vi "Firmware Wizard.vi"() -> ()   [LabVIEW 2011, in "LMH-LINX.lvlib"]
doc: "Wizard for uploading firmware to LINX devices."
uses:
  vi.lib/MakerHub/LINX/LMH-LINX.lvlib
  vi.lib/MakerHub/LINX/Private/Type Defs/Device Family.ctl
  vi.lib/MakerHub/LINX/Private/Type Defs/Devices/Device Type.ctl
  vi.lib/MakerHub/LINX/Private/Device/Type Defs/Wifi Config.ctl
  vi.lib/MakerHub/LINX/Private/Type Defs/WIFI Security Type.ctl
  vi.lib/MakerHub/LINX/Private/Type Defs/Deploy Firmware State.ctl
  vi.lib/MakerHub/LINX/Private/Type Defs/All Firmware Data FGV States.ctl
  vi.lib/MakerHub/LINX/Private/Device/Type Defs/Firmware Interface.ctl
  vi.lib/MakerHub/LINX/Private/Device/Type Defs/TCP Config.ctl
  <vilib>/MakerHub/Toolbox/LMH-Toolbox.lvlib
  vi.lib/MakerHub/LINX/Private/Device/Device.lvlib
panel:
  out "Error Out":errorcluster
  out "Log Path":path
  in  "Device Family Enum":T1 items=["National Instruments", "Digilent", "Arduino"]
  in  "Error In":errorcluster
  out "Tab Control":T2(tab)=enum."Device"
  in  "Firmware Available?":string
  in  "Settings Button":bool
  out "Device Image":picture
  in  "Device Help":bool
  in  "Device Type":T3 items=["Arduino Leonardo", "Arduino Mega2560", "Arduino Nano", "Arduino Pro Micro", "Arduino Uno"]
  in  "Device Family":T1 items=["Arduino", "Digilent", "PJRC", "Sparkfun"]
  in  "Device Cancel":bool
  in  "Device Next":bool
  in  "Firmware Program Interface":u16(ring) items=["Serial / USB"]
  in  "Config Message":string
  in  "Int Help":bool
  in  "Int Previous":bool
  in  "Int Cancel":bool
  in  "Int Next":bool
  out "Interface Config":enum32{"N/A", "Serial / USB", "USB", "TCP"}(tab)=enum."Serial / USB"
  in  "Upload COM Port":refnum<visa-resource-name>="ASRL1::INSTR"
  out "Firmware Configuration":enum32{"Serial", "Ethernet", "WIFI"}(tab)=enum."WIFI"
  in  "Port":u16=927
  in  "IP Address":string="192.168.1.27"
  in  "Wifi Configuration":T4
  in  "Firmware Description":string
  in  "FWV Help":bool
  in  "FWV Cancel":bool
  in  "FWV Next":bool
  in  "FWV Previous":bool
  in  "Firmware Version":u16(ring) items=["LINX - Serial / USB"]
  out "Deploy Progress Note":string
  in  "Deploy  Progress Bar":u8(slide) scale=0.0..100.0
  in  "View Log":bool
  in  "LINX Forum Link":string="www.labviewhacker.com/forums/linx"
  in  "LINX Landing Page Link":string="www.labviewhacker.com/linx"
  in  "Summary Launch Example":bool
  in  "Summary Text":string
  in  "Summary Next":bool
  in  "Summary Help":bool
  # "Ethernet Settings"
  # "WIFI Settings"
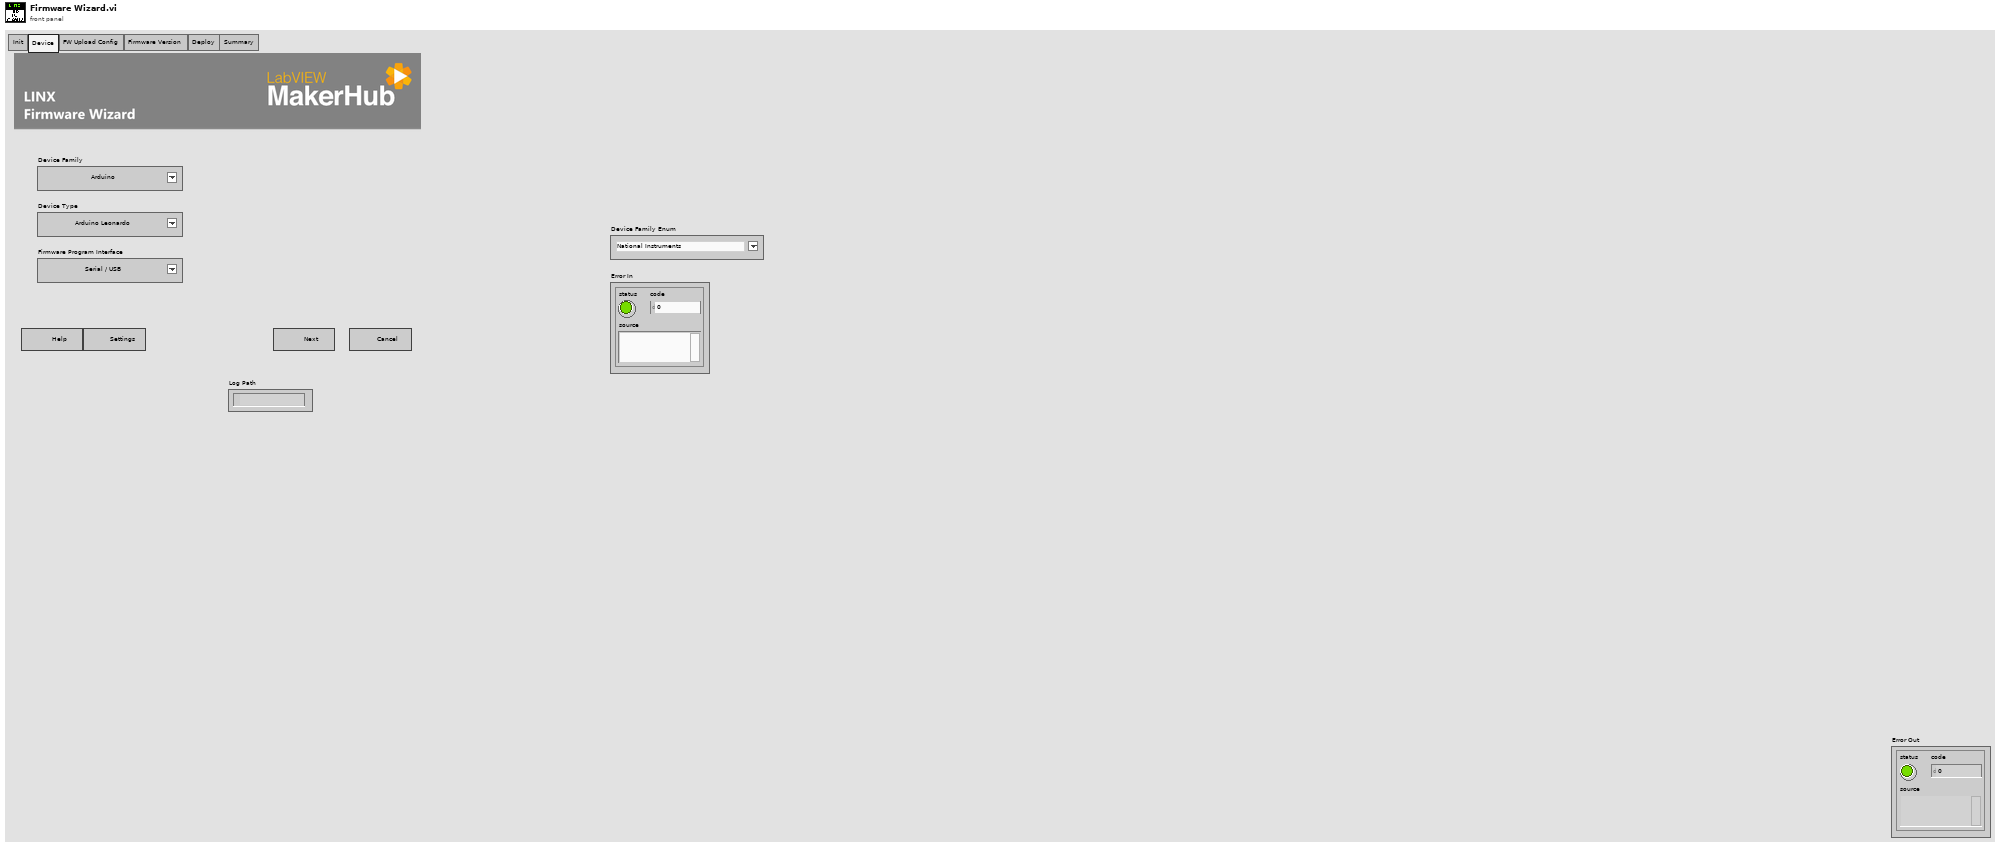
[diagram p1: front panel]
types:
  T1 = typedef "LMH-LINX.lvlib/Device Family.ctl" = u16
  T2 = enum32{"Init", "Device", "FW Upload Config", "Firmware Version", "Deploy", "Summary"}
  T3 = typedef "LMH-LINX.lvlib/Device Type.ctl" = u16
  T4 = typedef "LMH-LINX.lvlib/Device.lvlib/Wifi Config.ctl" = cluster{"SSID":string, "IP Address":string, "Port":u16, "WIFI Security Type":T5, "Password":string}
  T5 = typedef "LMH-LINX.lvlib/WIFI Security Type.ctl" = enum8{"None", "WPA2 Password", "WPA2 Key", "WEP40", "WEP104"}
  T6 = enum32{"invalid OS target", "Mac OS", "Windows 3.1", "Windows 95/NT", "Solaris 1", "Solaris 2", "HP-UX", "PowerMAX", "Linux", "Irix", "Rhapsody", "BeOS", "AIX", "OSF1", "VxWorks", "PharLap", "Carbon", "RTX", "Windows x64", "Linux x64"}
  T7 = typedef "LMH-LINX.lvlib/Deploy Firmware State.ctl" = enum32{"Init", "Device", "FW Upload Config", "Firmware Version", "Deploy", "Summary"}
  T8 = typedef "LMH-LINX.lvlib/All Firmware Data FGV States.ctl" = enum16{"Set", "Get"}
  T9 = enum8{"Enabled", "Disabled", "Disabled and Grayed Out"}
  T10 = typedef "LMH-LINX.lvlib/Firmware Interface.ctl" = enum32{"Serial ", "Ethernet", "WIFI"}
  T11 = typedef "LMH-LINX.lvlib/Device.lvlib/TCP Config.ctl" = cluster{"IP Address":string, "Port":u16}
  T12 = typedef "LMH-LINX.lvlib/Device Firmware.ctl" = cluster{"Firmware Name":string, "Firmware Path":path, "Description":string, "LINX Interface":string, "Flash Util Working Dir":path, "Flash Util Name":string, "Flash Util Args":string, "Flash Timeout (ms)":i32}
  T13 = enum16{"Left Button", "Center Button", "Right Button", "Window Close"}
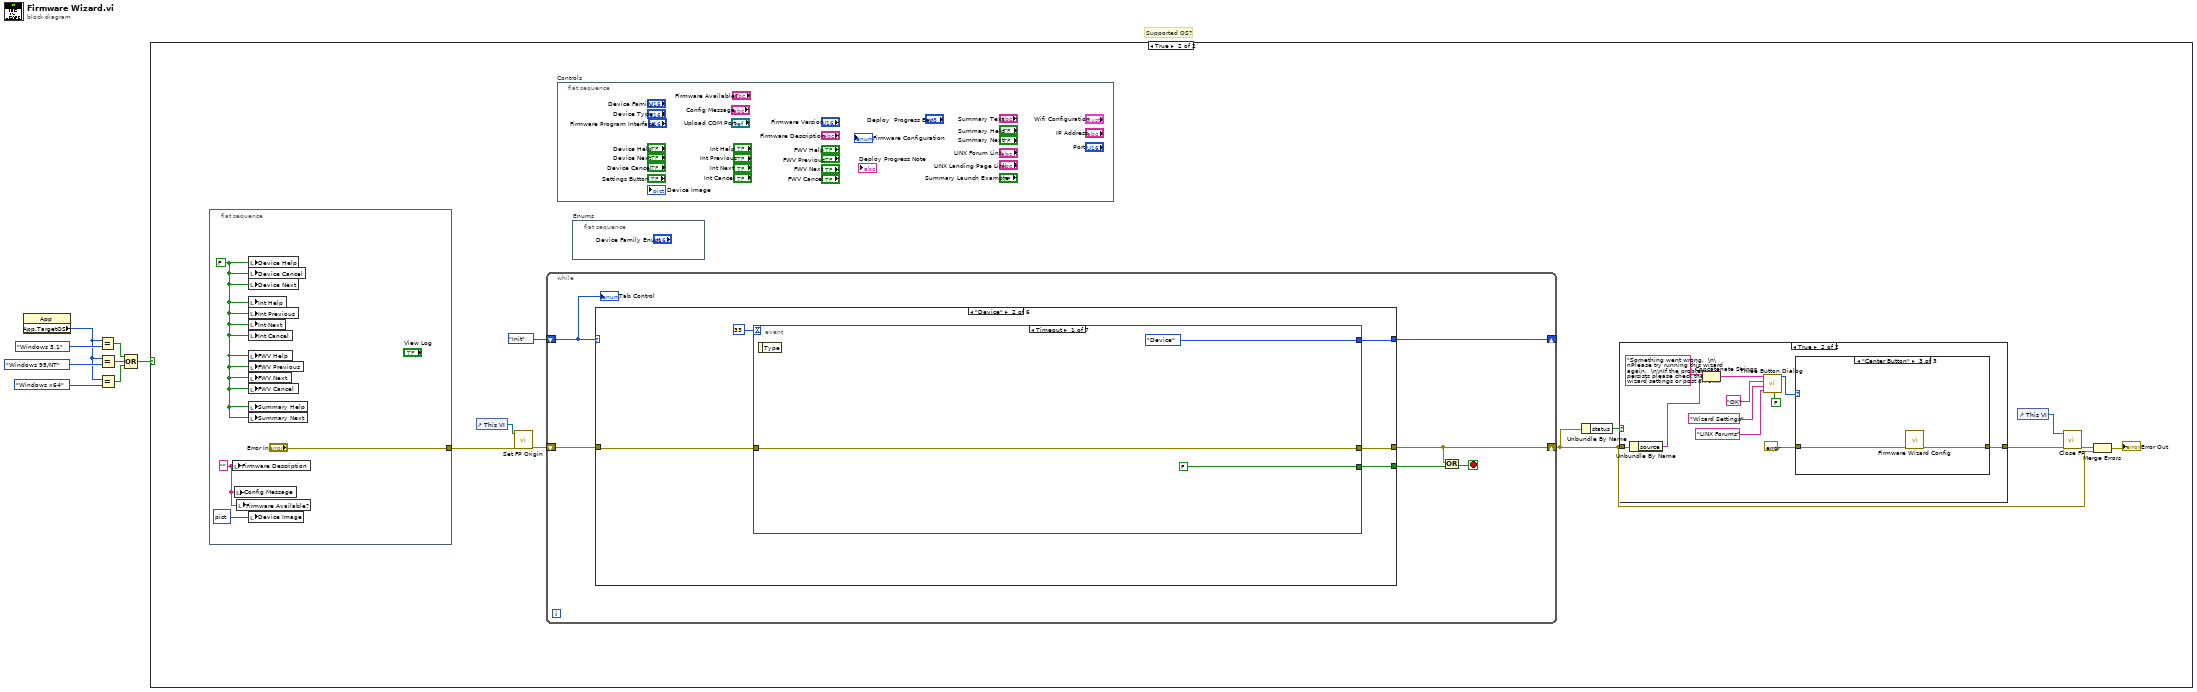
[diagram p0: block diagram]
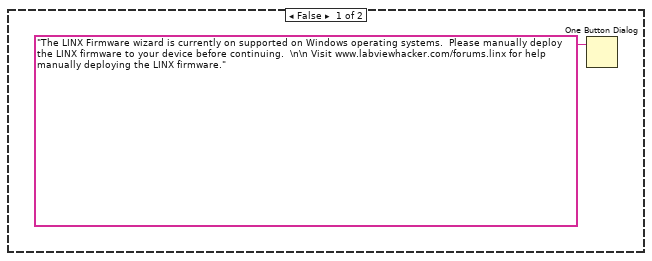
[diagram p2: hidden frame]
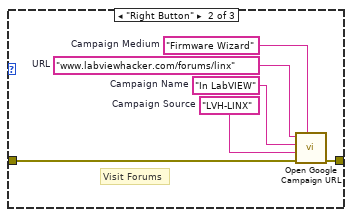
[diagram p5: hidden frame]
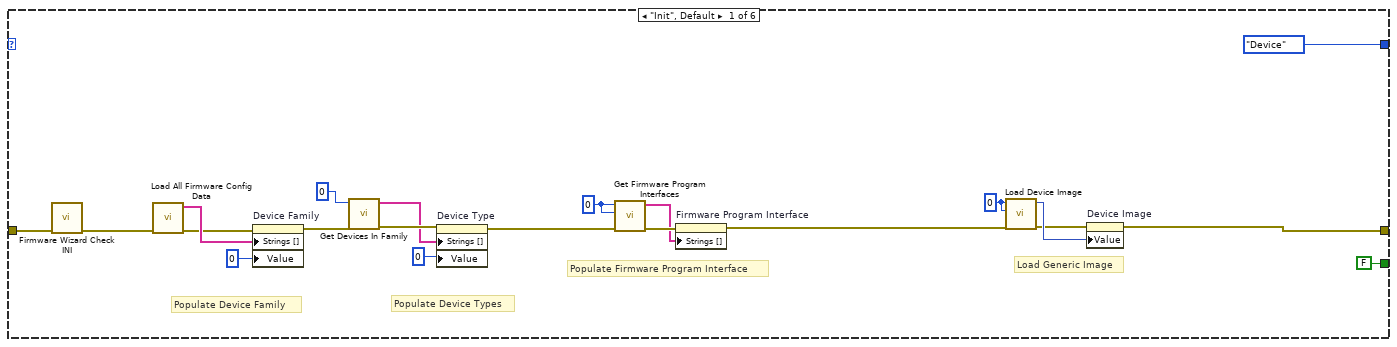
[diagram p6: hidden frame]
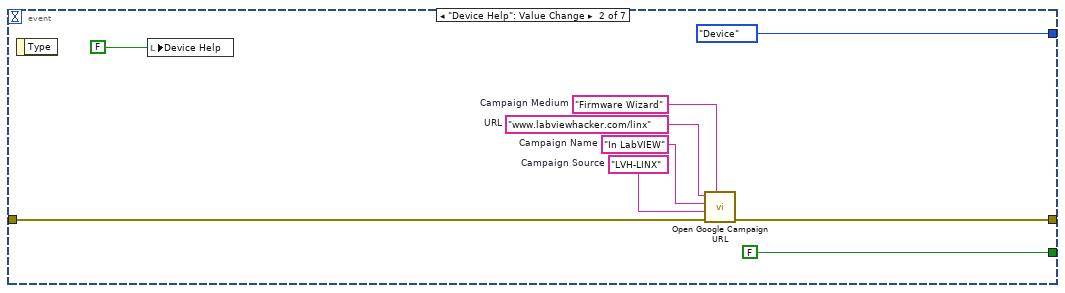
[diagram p7: hidden frame]
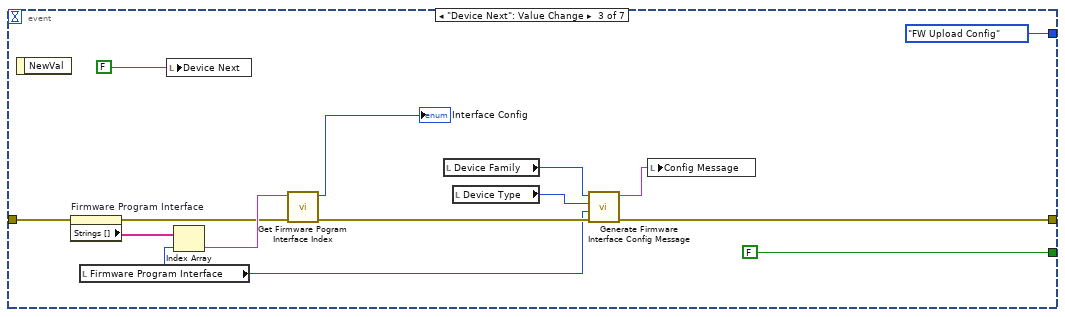
[diagram p8: hidden frame]
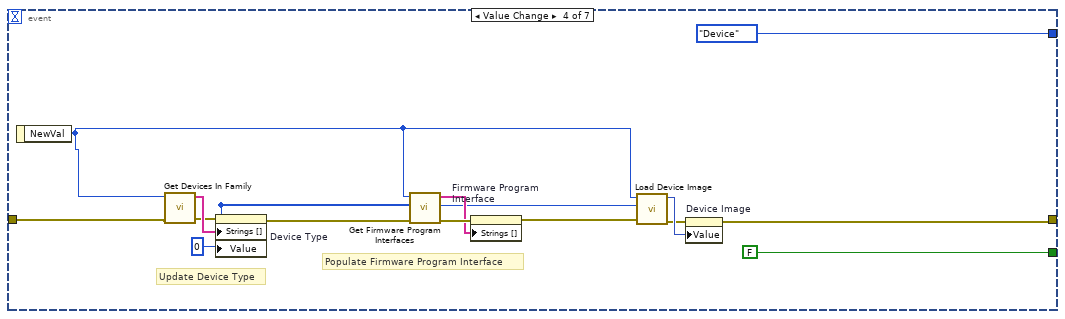
[diagram p9: hidden frame]
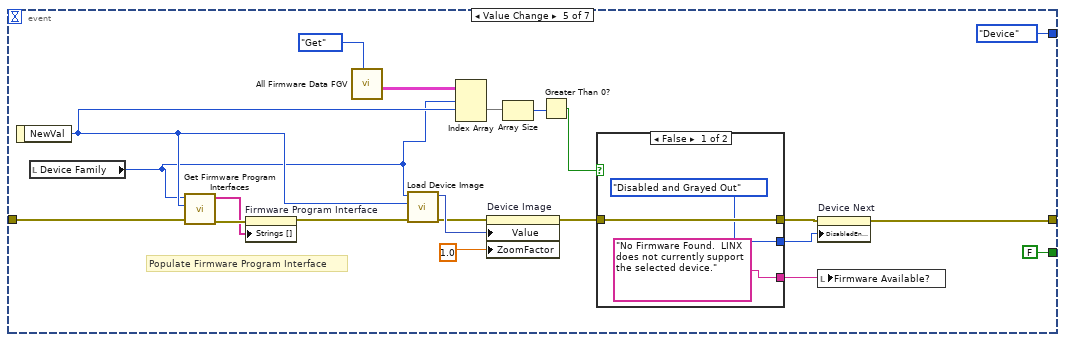
[diagram p10: hidden frame]
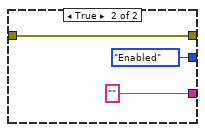
[diagram p11: hidden frame]
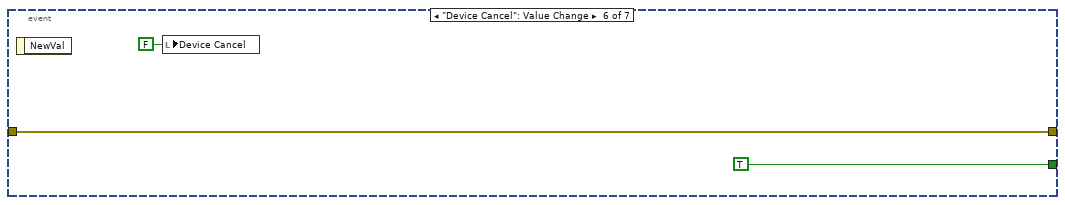
[diagram p12: hidden frame]
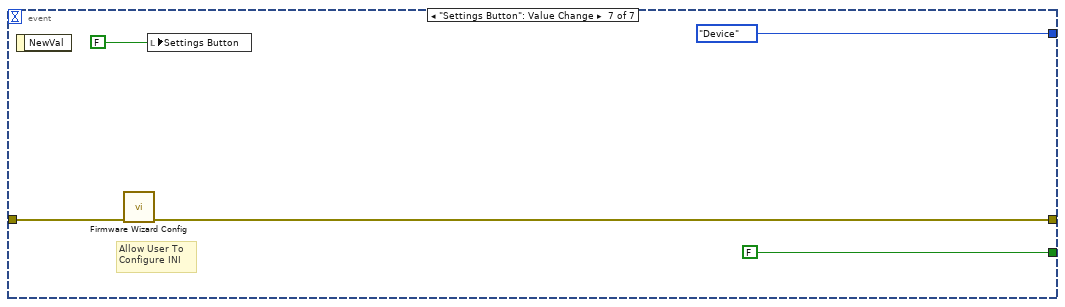
[diagram p13: hidden frame]
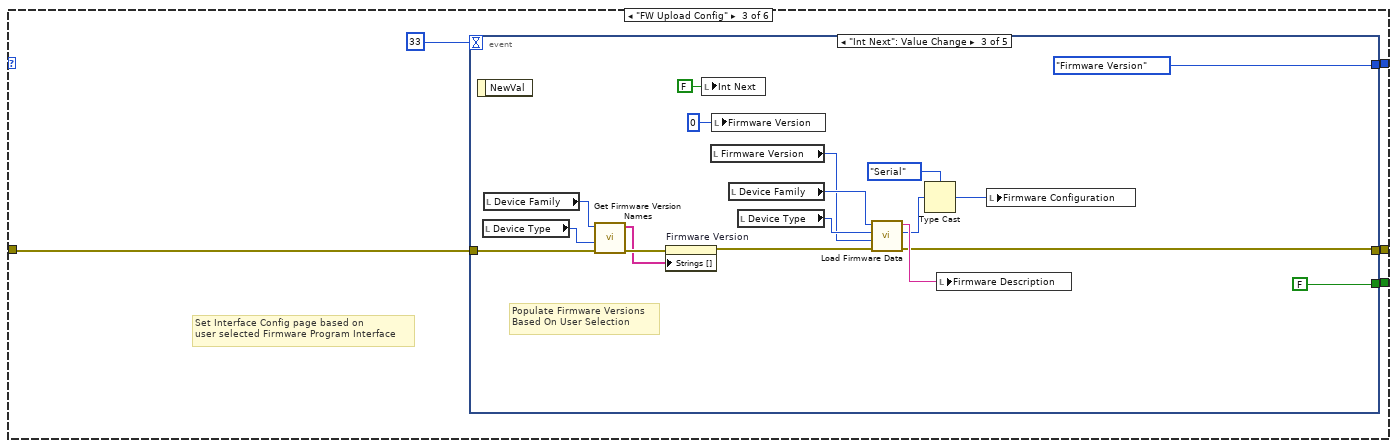
[diagram p14: hidden frame]
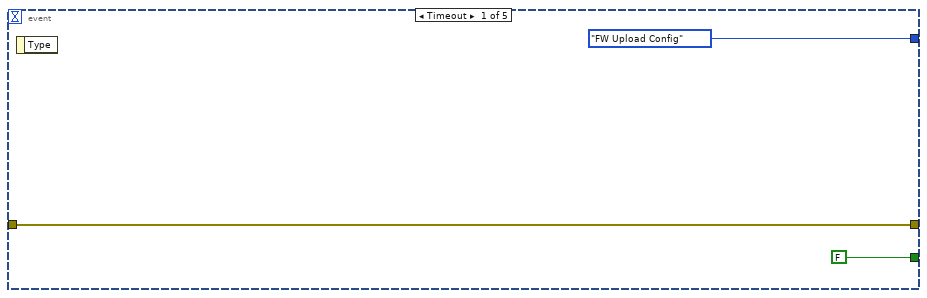
[diagram p15: hidden frame]
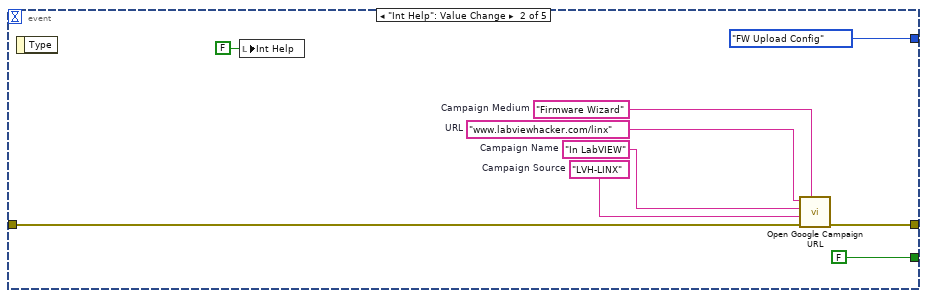
[diagram p16: hidden frame]
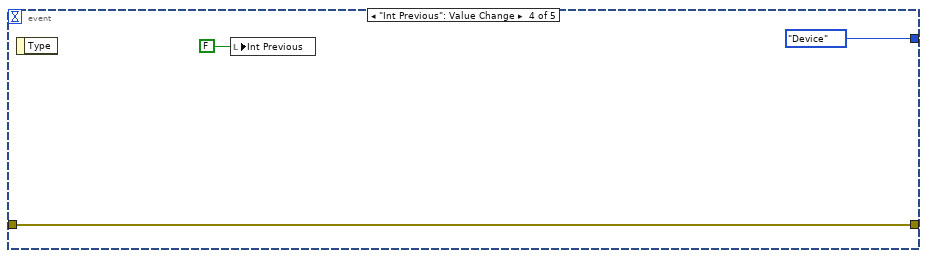
[diagram p17: hidden frame]
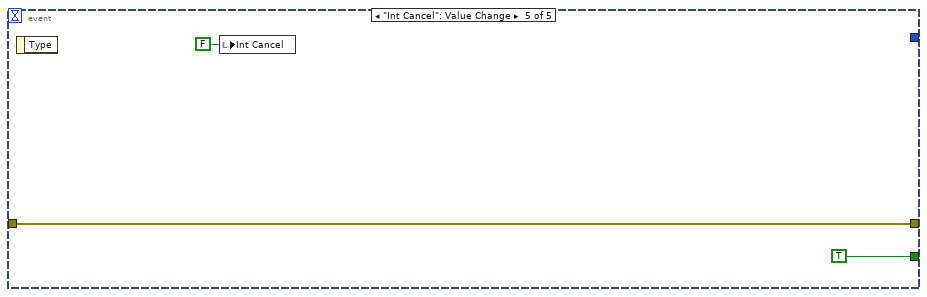
[diagram p18: hidden frame]
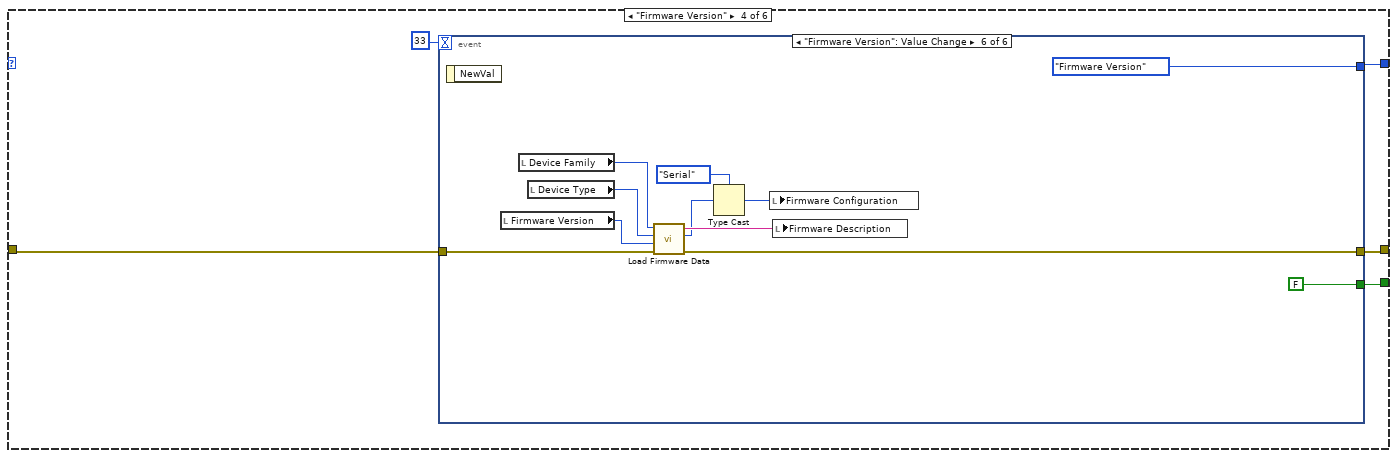
[diagram p19: hidden frame]
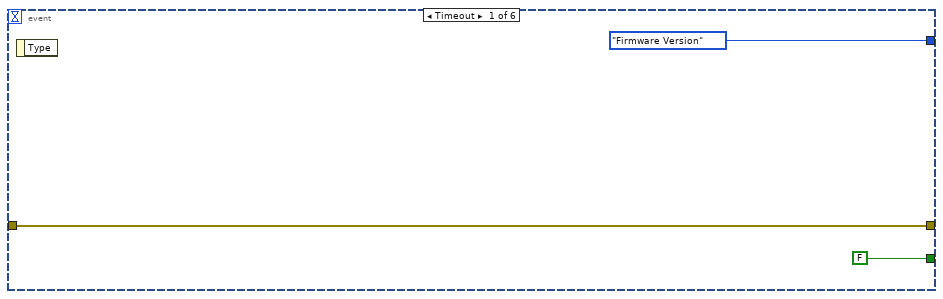
[diagram p20: hidden frame]
diagram:
  # "Supported OS?"
  n1 = property class="App"() -> ("App.TargetOS"=w6:T6)  [unwired: 2 in, 2 out]
  n2 = Equal?(x=w6, y=T6."Windows 3.1" ("Application:Target:Operating System")) -> (x = y?=w4:bool)
  n3 = Equal?(x=w6, y=T6."Windows 95/NT" ("Application:Target:Operating System")) -> (x = y?=w3:bool)
  n4 = Equal?(x=w6, y=T6."Windows x64" ("Application:Target:Operating System")) -> (x = y?=w2:bool)
  n5 = Compound Arithmetic op=OR(w4, w3, w2) -> (w1:bool)
  n6 = case shown="True" w1 {
    frame False {
      n7 = One Button Dialog(message="The LINX Firmware wizard is currently on supported on Windows operating systems.  Please manually deploy the LINX firmware to your device before continuing.  \n\n Visit www.labviewhacker.com/forums.linx for help manually deploying the LINX firmware.") -> ()  [unwired: 1 in, 1 out]
    }
    frame True {
      n8 = flat-sequence {
        tunnel: ["Error In"] -> w17
        frame #0 {
          w42 = "" ("Firmware Description")
          w44 = FALSE ("Cancel")
          n9 = local write "Firmware Description"(w42) -> ()
          n10 = local write "Config Message"(w42) -> ()
          n11 = local write "Firmware Available?"(w42) -> ()
          n12 = local write "Device Help"(w44) -> ()
          n13 = local write "Device Cancel"(w44) -> ()
          n14 = local write "Device Next"(w44) -> ()
          n15 = local write "Int Help"(w44) -> ()
          n16 = local write "Int Previous"(w44) -> ()
          n17 = local write "Int Next"(w44) -> ()
          n18 = local write "Int Cancel"(w44) -> ()
          n19 = local write "FWV Help"(w44) -> ()
          n20 = local write "FWV Previous"(w44) -> ()
          n21 = local write "FWV Next"(w44) -> ()
          n22 = local write "FWV Cancel"(w44) -> ()
          n23 = local write "Summary Help"(w44) -> ()
          n24 = local write "Summary Next"(w44) -> ()
          n25 = local write "Device Image"(picture data[5B] ("2D Picture")) -> ()
        }
      }
      n26 = control-ref of="This VI"() -> (w18:refnum<vi>)
      n27 = call <vilib>:"Set FP Origin.vi"("Error In"=w17, "VI Ref"=w18) -> ("Error Out"=w16:errorcluster)  [unwired: 9 in]
      n28 = while {
        shift-right: [w48] -> _
        shift-left: Deploy_Firmware_State."Init" ("Deploy Firmware State") -> [w50]
        shift-right: [w47] -> w11
        shift-left: w16 -> [w49]
        stop <- w46 stop-if-true
        n29 = case shown="\"Device\"" w50 {
          tunnel: [w61 w75 w155 w197 w233 w274] -> w47
          tunnel: w49 -> [w53 w74 w152 w196 w237 w270]
          tunnel: [Deploy_Firmware_State."Device" ("Deploy Firmware State") w73 w156 w194 Deploy_Firmware_State."Summary" ("Deploy Firmware State") w272] -> w48
          tunnel: [FALSE w72 w153 w193 FALSE w271] -> w45
          frame "Init", Default {
            w54 = 0 ("Device Family Index")
            w65 = 0 ("Device Family")
            # "Load Generic Image"
            # "Populate Firmware Program Interface"
            # "Populate Device Types"
            # "Populate Device Family"
            n30 = call "Firmware Wizard Check INI.vi"("Error In"=w53) -> ("Error Out"=w52:errorcluster)  [unwired: 10 in]
            n31 = call "Load All Firmware Config Data.vi"("Error In"=w52) -> ("Error Out"=w55:errorcluster, "Families"=w56:string[])  [unwired: 7 in, 2 out]
            n32 = property on="Device Family" class="Ring (strict)"(error in=w55, "Strings []"=w56, "Value"=u16 0 ("Device Family")) -> (error out=w60:errorcluster)  [unwired: 1 in, 1 out]
            n33 = call "Get Devices In Family.vi"("Error In"=w60, "Family Index"=0 ("Device Family")) -> ("Error Out"=w59:errorcluster, "Devices"=w58:string[])  [unwired: 8 in]
            n34 = property on="Device Type" class="Ring (strict)"(error in=w59, "Strings []"=w58, "Value"=u16 0 ("Device Family")) -> (error out=w66:errorcluster)  [unwired: 1 in, 1 out]
            n35 = call "Get Firmware Program Interfaces.vi"("Error In"=w66, "Device Index"=w65, "Family Index"=w65) -> ("Error Out"=w68:errorcluster, "Firmware Program Interfaces"=w67:string[])  [unwired: 7 in]
            n36 = property on="Firmware Program Interface" class="Ring (strict)"(error in=w68, "Strings []"=w67) -> (error out=w51:errorcluster)  [unwired: 1 in, 1 out]
            n37 = call "Load Device Image.vi"("Error In"=w51, "Device Index"=w54, "Device Family Index"=w54) -> ("Error Out"=w62:errorcluster, "Device Image"=w63:picture)  [unwired: 6 in, 1 out]
            n38 = property on="Device Image" class="Pict"(error in=w62, "Value"=w63) -> (error out=w61:errorcluster)  [unwired: 1 in, 1 out]
          }
          frame "Device" {
            n39 = event shown="[0] Timeout" {
              selector: _ -> [_ _ _ _ _ _ _]
              dyn-events: _ -> [_ _ _ _ _ _ _]
              timeout: 33 -> [_ _ _ _ _ _ _]
              tunnel: [w79 w82 w99 w108 w126 w145 w148] -> w75
              tunnel: w74 -> [w79 w81 w95 w107 w137 w145 w149]
              tunnel: [Deploy_Firmware_State."Device" ("Deploy Firmware State") Deploy_Firmware_State."Device" ("Deploy Firmware State") Deploy_Firmware_State."FW Upload Config" ("Deploy Firmware State") Deploy_Firmware_State."Device" ("Deploy Firmware State") Deploy_Firmware_State."Device" ("Deploy Firmware State") _ Deploy_Firmware_State."Device" ("Deploy Firmware State")] -> w73
              tunnel: [FALSE FALSE FALSE FALSE FALSE TRUE FALSE] -> w72
              event Timeout {
                n40 = event-data() -> ()  [unwired: 1 in, 1 out]
              }
              event "Device Help": Value Change {
                w80 = "LVH-LINX"  # Campaign Source
                w83 = "In LabVIEW"  # Campaign Name
                w84 = "Firmware Wizard"  # Campaign Medium
                w85 = "www.labviewhacker.com/linx"  # URL
                n41 = event-data() -> ()  [unwired: 1 in, 1 out]
                n42 = local write "Device Help"(FALSE ("Device Help")) -> ()
                n43 = call <vilib>:"Open Google Campaign URL.vi"("Campaign Medium"=w84, "Error In"=w81, "Campaign Source"=w80, "Campaign Name"=w83, "URL"=w85) -> ("Error Out"=w82:errorcluster)  [unwired: 5 in, 1 out]
              }
              event "Device Next": Value Change {
                n44 = event-data() -> ()  [unwired: 1 in, 1 out]
                n45 = property on="Firmware Program Interface" class="Ring (strict)"(error in=w95) -> (error out=w96:errorcluster, "Strings []"=w98:string[])  [unwired: 1 in, 1 out]
                n46 = local read "Firmware Program Interface"() -> (w90:u16)
                n47 = local write "Device Next"(FALSE ("Next")) -> ()
                n48 = Index Array(array=w98, index=w90) -> (element=w97:string)
                n49 = call "Get Firmware Pogram Interface Index.vi"("Error In"=w96, "Firmware Program Interface"=w97) -> ("Error Out"=w94:errorcluster, "Interface Index"=→"Interface Config":i32)  [unwired: 8 in]
                n50 = local read "Device Family"() -> (w92:T1)
                n51 = local read "Device Type"() -> (w91:T3)
                n52 = call "Generate Firmware Interface Config Message.vi"("Error In"=w94, "Firmware Program Interface Index"=w90, "Device Index"=w91, "Family Index"=w92) -> ("Error Out"=w99:errorcluster, "Config Message"=w100:string)  [unwired: 6 in]
                n53 = local write "Config Message"(w100) -> ()
              }
              event Value Change {
                w103 = u16 0 ("Device Family")
                # "Populate Firmware Program Interface"
                # "Update Device Type"
                n54 = event-data() -> ("NewVal"=w104:T1)  [unwired: 1 in]
                n55 = call "Get Devices In Family.vi"("Error In"=w107, "Family Index"=w104) -> ("Error Out"=w105:errorcluster, "Devices"=w106:string[])  [unwired: 8 in]
                n56 = property on="Device Type" class="Ring (strict)"(error in=w105, "Strings []"=w106, "Value"=w103) -> (error out=w113:errorcluster)  [unwired: 1 in, 1 out]
                n57 = call "Get Firmware Program Interfaces.vi"("Error In"=w113, "Device Index"=w103, "Family Index"=w104) -> ("Error Out"=w115:errorcluster, "Firmware Program Interfaces"=w114:string[])  [unwired: 7 in]
                n58 = property on="Firmware Program Interface" class="Ring (strict)"(error in=w115, "Strings []"=w114) -> (error out=w109:errorcluster)  [unwired: 1 in, 1 out]
                n59 = call "Load Device Image.vi"("Error In"=w109, "Device Index"=w103, "Device Family Index"=w104) -> ("Error Out"=w110:errorcluster, "Device Image"=w111:picture)  [unwired: 6 in, 1 out]
                n60 = property on="Device Image" class="Pict"(error in=w110, "Value"=w111) -> (error out=w108:errorcluster)  [unwired: 1 in, 1 out]
              }
              event Value Change {
                # "Populate Firmware Program Interface"
                n61 = event-data() -> ("NewVal"=w118:T3)  [unwired: 1 in]
                n62 = local read "Device Family"() -> (w117:T1)
                n63 = call "Get Firmware Program Interfaces.vi"("Error In"=w137, "Device Index"=w118, "Family Index"=w117) -> ("Error Out"=w136:errorcluster, "Firmware Program Interfaces"=w135:string[])  [unwired: 7 in]
                n64 = property on="Firmware Program Interface" class="Ring (strict)"(error in=w136, "Strings []"=w135) -> (error out=w132:errorcluster)  [unwired: 1 in, 1 out]
                n65 = call "All Firmware Data FGV.vi"("All Firmware Data FGV States"=All_Firmware_Data_FGV_States."Get") -> ("Firmwares"=w123:T12[][][])  [unwired: 7 in, 3 out]
                n66 = call "Load Device Image.vi"("Error In"=w132, "Device Index"=w118, "Device Family Index"=w117) -> ("Error Out"=w129:errorcluster, "Device Image"=w131:picture)  [unwired: 6 in, 1 out]
                n67 = Index Array(array=w123, index (dim 0)=w117, index (dim 1)=w118) -> (element=w122:T12[])  [unwired: 1 in]
                n68 = property on="Device Image" class="Pict"(error in=w129, "Value"=w131, "ZoomFactor"=sgl 1.0 ("Zoom Factor")) -> (error out=w128:errorcluster)  [unwired: 1 in, 1 out]
                n69 = Array Size(array=w122) -> (size(s)=w121:i32)
                n70 = Greater Than 0?(x=w121) -> (x > 0?=w120:bool)
                n71 = case shown="False" w120 {
                  tunnel: [w140 w143] -> w127
                  tunnel: w128 -> [w140 w143]
                  tunnel: [T9."Disabled and Grayed Out" ("Disabled") T9."Enabled" ("Disabled")] -> w125
                  tunnel: ["No Firmware Found.  LINX does not currently support the selected device." ("Firmware Available?") "" ("Firmware Available?")] -> w124
                  frame False {
                  }
                  frame True {
                  }
                }
                n72 = property on="Device Next" class="Bool (strict)"(error in=w127, "DisabledEnum"=w125) -> (error out=w126:errorcluster)  [unwired: 1 in, 1 out]
                n73 = local write "Firmware Available?"(w124) -> ()
              }
              event "Device Cancel": Value Change {
                n74 = event-data() -> ()  [unwired: 1 in, 1 out]
                n75 = local write "Device Cancel"(FALSE ("Device Cancel")) -> ()
              }
              event "Settings Button": Value Change {
                # "Allow User To \nConfigure INI"
                n76 = event-data() -> ()  [unwired: 1 in, 1 out]
                n77 = call "Firmware Wizard Config.vi"("Error In"=w149) -> ("Error Out"=w148:errorcluster)  [unwired: 10 in]
                n78 = local write "Settings Button"(FALSE ("Settings Button")) -> ()
              }
            }
          }
          frame "FW Upload Config" {
            # "Set Interface Config page based on \nuser selected Firmware Program Interface"
            n79 = event shown="[2] \"Int Next\": Value Change" {
              selector: _ -> [_ _ _ _ _]
              dyn-events: _ -> [_ _ _ _ _]
              timeout: 33 -> [_ _ _ _ _]
              tunnel: [Deploy_Firmware_State."FW Upload Config" ("Deploy Firmware State") Deploy_Firmware_State."FW Upload Config" ("Deploy Firmware State") Deploy_Firmware_State."Firmware Version" ("Deploy Firmware State") Deploy_Firmware_State."Device" ("Deploy Firmware State") _] -> w156
              tunnel: [w158 w160 w173 w189 w190] -> w155
              tunnel: w152 -> [w158 w161 w186 w189 w190]
              tunnel: [FALSE FALSE FALSE _ TRUE] -> w153
              event Timeout {
                n80 = event-data() -> ()  [unwired: 1 in, 1 out]
              }
              event "Int Help": Value Change {
                w162 = "LVH-LINX"  # Campaign Source
                w163 = "In LabVIEW"  # Campaign Name
                w164 = "Firmware Wizard"  # Campaign Medium
                w165 = "www.labviewhacker.com/linx"  # URL
                n81 = event-data() -> ()  [unwired: 1 in, 1 out]
                n82 = local write "Int Help"(FALSE ("Int Help")) -> ()
                n83 = call <vilib>:"Open Google Campaign URL.vi"("Campaign Medium"=w164, "Error In"=w161, "Campaign Source"=w162, "Campaign Name"=w163, "URL"=w165) -> ("Error Out"=w160:errorcluster)  [unwired: 5 in, 1 out]
              }
              event "Int Next": Value Change {
                # "Populate Firmware Versions\nBased On User Selection"
                n84 = event-data() -> ()  [unwired: 1 in, 1 out]
                n85 = local read "Device Type"() -> (w183:T3)
                n86 = local read "Device Family"() -> (w182:T1)
                n87 = call "Get Firmware Version Names.vi"("Error In"=w186, "Device Index"=w183, "Family Index"=w182) -> ("Error Out"=w185:errorcluster, "Firmware Version Names"=w184:string[])  [unwired: 6 in, 1 out]
                n88 = property on="Firmware Version" class="Ring (strict)"(error in=w185, "Strings []"=w184) -> (error out=w177:errorcluster)  [unwired: 1 in, 1 out]
                n89 = local write "Int Next"(FALSE ("Int Next")) -> ()
                n90 = local read "Firmware Version"() -> (w170:u16)
                n91 = local write "Firmware Version"(0) -> ()
                n92 = local read "Device Family"() -> (w172:T1)
                n93 = local read "Device Type"() -> (w171:T3)
                n94 = call "Load Firmware Data.vi"("Error In"=w177, "Firmware Index"=w170, "Device Index"=w171, "Family Index"=w172) -> ("Error Out"=w173:errorcluster, "Firmware Interface"=w169:T10, "Firmware Description"=w178:string)  [unwired: 5 in]
                n95 = Type Cast(type=enum32{"Serial", "Ethernet", "WIFI"}."Serial" ("Firmware Configuration"), x=w169) -> (*(type *) &x=w174:enum32{"Serial", "Ethernet", "WIFI"})
                n96 = local write "Firmware Description"(w178) -> ()
                n97 = local write "Firmware Configuration"(w174) -> ()
              }
              event "Int Previous": Value Change {
                n98 = event-data() -> ()  [unwired: 1 in, 1 out]
                n99 = local write "Int Previous"(FALSE ("Previous")) -> ()
              }
              event "Int Cancel": Value Change {
                n100 = event-data() -> ()  [unwired: 1 in, 1 out]
                n101 = local write "Int Cancel"(FALSE ("Int Cancel")) -> ()
              }
            }
          }
          frame "Firmware Version" {
            n102 = event shown="[5] \"Firmware Version\": Value Change" {
              selector: _ -> [_ _ _ _ _ _]
              dyn-events: _ -> [_ _ _ _ _ _]
              timeout: 33 -> [_ _ _ _ _ _]
              tunnel: [w200 w202 w212 w216 w220 w229] -> w197
              tunnel: w196 -> [w200 w201 w212 w216 w220 w230]
              tunnel: [Deploy_Firmware_State."Firmware Version" ("Deploy Firmware State") Deploy_Firmware_State."Firmware Version" ("Deploy Firmware State") Deploy_Firmware_State."FW Upload Config" ("Deploy Firmware State") Deploy_Firmware_State."Deploy" ("Deploy Firmware State") Deploy_Firmware_State."Init" ("Deploy Firmware State") Deploy_Firmware_State."Firmware Version" ("Deploy Firmware State")] -> w194
              tunnel: [FALSE FALSE FALSE FALSE TRUE FALSE] -> w193
              event Timeout {
                n103 = event-data() -> ()  [unwired: 1 in, 1 out]
              }
              event "FWV Help": Value Change {
                w203 = "LVH-LINX"  # Campaign Source
                w204 = "In LabVIEW"  # Campaign Name
                w205 = "Firmware Wizard"  # Campaign Medium
                w206 = "www.labviewhacker.com/linx"  # URL
                n104 = event-data() -> ()  [unwired: 1 in, 1 out]
                n105 = local write "FWV Help"(FALSE ("FWV Help")) -> ()
                n106 = call <vilib>:"Open Google Campaign URL.vi"("Campaign Medium"=w205, "Error In"=w201, "Campaign Source"=w203, "Campaign Name"=w204, "URL"=w206) -> ("Error Out"=w202:errorcluster)  [unwired: 5 in, 1 out]
              }
              event "FWV Previous": Value Change {
                n107 = event-data() -> ()  [unwired: 1 in, 1 out]
                n108 = local write "FWV Previous"(FALSE ("FWV Previous")) -> ()
              }
              event "FWV Next": Value Change {
                n109 = event-data() -> ()  [unwired: 1 in, 1 out]
                n110 = local write "FWV Next"(FALSE ("FWV Previous")) -> ()
              }
              event "FWV Cancel": Value Change {
                n111 = event-data() -> ()  [unwired: 1 in, 1 out]
                n112 = local write "FWV Cancel"(FALSE ("FWV Previous")) -> ()
              }
              event "Firmware Version": Value Change {
                n113 = event-data() -> ()  [unwired: 1 in, 1 out]
                n114 = local read "Firmware Version"() -> (w222:u16)
                n115 = local read "Device Family"() -> (w224:T1)
                n116 = local read "Device Type"() -> (w223:T3)
                n117 = call "Load Firmware Data.vi"("Error In"=w230, "Firmware Index"=w222, "Device Index"=w223, "Family Index"=w224) -> ("Error Out"=w229:errorcluster, "Firmware Interface"=w226:T10, "Firmware Description"=w228:string)  [unwired: 5 in]
                n118 = Type Cast(type=enum32{"Serial", "Ethernet", "WIFI"}."Serial" ("Firmware Configuration"), x=w226) -> (*(type *) &x=w225:enum32{"Serial", "Ethernet", "WIFI"})
                n119 = local write "Firmware Configuration"(w225) -> ()
                n120 = local write "Firmware Description"(w228) -> ()
              }
            }
          }
          frame "Deploy" {
            n121 = flat-sequence {
              tunnel: w237 -> [w242]
              tunnel: [w242] -> w236
              tunnel: [w248] -> w239
              tunnel: [w247] -> w238
              tunnel: w236 -> [w246]
              tunnel: w239 -> [w253]
              tunnel: w238 -> [w252]
              tunnel: [w253] -> w235
              tunnel: [w252] -> w234
              tunnel: w235 -> [w262]
              tunnel: w234 -> [w261]
              tunnel: [w256] -> w233
              frame #0 {
                n122 = local write "Deploy Progress Note"("Uploading Device Firmware" ("Deploy Progress Note")) -> ()
              }
              frame #1 {
                n123 = local read "Firmware Version"() -> (w245:u16)
                n124 = local read "Upload COM Port"() -> (w247:refnum<visa-resource-name>)
                n125 = local read "Device Family"() -> (w250:T1)
                n126 = local read "Device Type"() -> (w249:T3)
                n127 = control-ref of="Deploy  Progress Bar"() -> (w251:refnum<vi>)
                n128 = call "Upload Firmware.vi"("Progress Bar"=w251, "COM Port"=w247, "Error In"=w246, "Firmware Index"=w245, "Device Index"=w249, "Family Index"=w250) -> ("Error Out"=w248:errorcluster, "Log Path"=→"Log Path":path)  [unwired: 4 in]
              }
              frame #2 {
                n129 = local write "Deploy Progress Note"("Configuring Device Settings" ("Deploy Progress Note")) -> ()
              }
              frame #3 {
                n130 = local read "Firmware Configuration"() -> (w258:enum32{"Serial", "Ethernet", "WIFI"})
                n131 = local read "IP Address"() -> (w265:string)
                n132 = local read "Port"() -> (w264:u16)
                n133 = local read "Wifi Configuration"() -> (w255:T4)
                n134 = Bundle By Name(cluster=T11 {"IP Address"="", "Port"=0} ("TCP Configuration"), "IP Address"=w265, "Port"=w264) -> (w260:T11)
                n135 = Type Cast(type=Firmware_Interface."Serial " ("Firmware Interface"), x=w258) -> (*(type *) &x=w259:T10)
                n136 = call "Configure LINX Device.vi"("Wifi Configuration"=w255, "TCP Configuration"=w260, "Error In"=w262, "Firmware Interface"=w259, "COM Port"=w261) -> ("Error Out"=w256:errorcluster)  [unwired: 6 in]
              }
            }
          }
          frame "Summary" {
            n137 = local read "Device Family"() -> (w268:T1)
            n138 = local read "Device Type"() -> (w267:T3)
            n139 = call "Generate Firmware Wizard Summary Message.vi"("Error In"=w270, "Device ID"=w267, "Device Family"=w268) -> ("Error Out"=w269:errorcluster, "Summary"=w266:string)  [unwired: 7 in]
            n140 = local write "Summary Text"(w266) -> ()
            n141 = event shown="[4] \"View Log\": Value Change" {
              selector: _ -> [_ _ _ _ _ _ _]
              dyn-events: _ -> [_ _ _ _ _ _ _]
              timeout: 33 -> [_ _ _ _ _ _ _]
              tunnel: [w277 w284 w291 w299 w300 w316 w339] -> w274
              tunnel: w269 -> [w277 w283 w290 w298 w301 w325 w339]
              tunnel: [Deploy_Firmware_State."Summary" ("Deploy Firmware State") Deploy_Firmware_State."Summary" ("Deploy Firmware State") Deploy_Firmware_State."Summary" ("Deploy Firmware State") Deploy_Firmware_State."Summary" ("Deploy Firmware State") Deploy_Firmware_State."Summary" ("Deploy Firmware State") Deploy_Firmware_State."Summary" ("Deploy Firmware State") Deploy_Firmware_State."Init" ("Deploy Firmware State")] -> w272
              tunnel: [FALSE _ _ _ _ TRUE TRUE] -> w271
              event Timeout {
                n142 = event-data() -> ()  [unwired: 1 in, 1 out]
              }
              event "LINX Forum Link": Mouse Down {
                w279 = "LVH-LINX"  # Campaign Source
                w280 = "In LabVIEW"  # Campaign Name
                w281 = "Firmware Wizard"  # Campaign Medium
                w282 = "www.labviewhacker.com/forums/linx"  # URL
                n143 = event-data() -> ()  [unwired: 1 in, 7 out]
                n144 = call <vilib>:"Open Google Campaign URL.vi"("Campaign Medium"=w281, "Error In"=w283, "Campaign Source"=w279, "Campaign Name"=w280, "URL"=w282) -> ("Error Out"=w284:errorcluster)  [unwired: 5 in, 1 out]
              }
              event "LINX Landing Page Link": Mouse Down {
                w286 = "LVH-LINX"  # Campaign Source
                w287 = "In LabVIEW"  # Campaign Name
                w288 = "Firmware Wizard"  # Campaign Medium
                w289 = "www.labviewhacker.com/linx"  # URL
                n145 = event-data() -> ()  [unwired: 1 in, 7 out]
                n146 = call <vilib>:"Open Google Campaign URL.vi"("Campaign Medium"=w288, "Error In"=w290, "Campaign Source"=w286, "Campaign Name"=w287, "URL"=w289) -> ("Error Out"=w291:errorcluster)  [unwired: 5 in, 1 out]
              }
              event "Summary Help": Value Change {
                w294 = "LVH-LINX"  # Campaign Source
                w295 = "In LabVIEW"  # Campaign Name
                w296 = "Firmware Wizard"  # Campaign Medium
                w297 = "www.labviewhacker.com/linx"  # URL
                n147 = event-data() -> ()  [unwired: 1 in, 1 out]
                n148 = local write "Summary Help"(FALSE ("Summary Help")) -> ()
                n149 = call <vilib>:"Open Google Campaign URL.vi"("Campaign Medium"=w296, "Error In"=w298, "Campaign Source"=w294, "Campaign Name"=w295, "URL"=w297) -> ("Error Out"=w299:errorcluster)  [unwired: 5 in, 1 out]
              }
              event "View Log": Value Change {
                w308 = "\"" ("string")
                # "Open Log File In Default Text Editor"
                n150 = event-data() -> ()  [unwired: 1 in, 5 out]
                n151 = local write "View Log"(FALSE ("Summary Help")) -> ()
                n152 = local read "Log Path"() -> (w303:path)
                n153 = Path To String(path=w303) -> (string=w309:string)
                n154 = Concatenate Strings("cmd /k" ("command line"), w308, w309, w308) -> (w306:string)
                n155 = call <vilib>:"System Exec.vi"("run minimized? (F)"=TRUE, "wait until completion? (T)"=FALSE, "command line"=w306) -> ("error out"=w302:errorcluster)  [unwired: 5 in, 3 out]
                n156 = Merge Errors(w302, w301) -> (w300:errorcluster)
              }
              event "Summary Launch Example": Value Change {
                n157 = event-data() -> ()  [unwired: 1 in, 1 out]
                n158 = local read "Firmware Configuration"() -> (w332:enum32{"Serial", "Ethernet", "WIFI"})
                n159 = call <vilib>:"Get Main Path.vi"("Error In"=w325) -> ("Error Out"=w326:errorcluster, "Main Dir"=w328:path)  [unwired: 8 in, 1 out]
                n160 = local write "Summary Launch Example"(FALSE ("Summary Launch Example")) -> ()
                n161 = call <vilib>:"Strip Path To Token.vi"("Error In"=w326, "Token (Regex)"="LabVIEW [0-9]+.?[0-9]?", "Path"=w328) -> ("Error Out"=w324:errorcluster, "Stripped Path"=w329:path)  [unwired: 6 in, 1 out]
                n162 = call <vilib>:"Append Relative Path String.vi"("Error In"=w324, "Relative Path"="\\examples\\MakerHub\\LINX", "Base Path"=w329) -> ("Error Out"=w315:errorcluster, "Absolute Path"=w314:path)  [unwired: 7 in]
                n163 = Type Cast(type=Firmware_Interface."Serial " ("Firmware Interface"), x=w332) -> (*(type *) &x=w330:T10)
                n164 = case shown="\"Ethernet\", \"WIFI\"" w330 {
                  tunnel: ["LINX - Blink (Simple).vi" ("name or relative path") "LINX - Blink (Simple) (TCP).vi" ("name or relative path")] -> w313
                  frame "Serial ", Default {
                  }
                  frame "Ethernet", "WIFI" {
                  }
                }
                n165 = Build Path(base path=w314, name or relative path=w313) -> (appended path=w322:path)
                n166 = Open VI Reference(vi path=w322, error in (no error)=w315) -> (vi reference=w321:refnum<vi>, error out=w320:errorcluster)  [unwired: 4 in]
                n167 = property class="VI"(reference=w321, error in=w320, "Front Panel.Open"=TRUE ("Front Panel Window:Open")) -> (reference out=w317:refnum<vi>, error out=w318:errorcluster)
                n168 = Close Reference(reference=w317, error in (no error)=w318) -> (error out=w316:errorcluster)
              }
              event "Summary Next": Value Change {
                n169 = event-data() -> ()  [unwired: 1 in, 1 out]
                n170 = local write "Summary Next"(FALSE ("FWV Previous")) -> ()
              }
            }
          }
        }
        n171 = Or(x=w47, y=w45) -> (x .or. y?=w46:bool)
        "Tab Control" <- w50
      }
      n172 = flat-sequence "Controls" {
        frame #0 {
        }
      }
      n173 = flat-sequence "Enums" {
        frame #0 {
        }
      }
      n174 = Unbundle By Name(w11) -> ("status"=w15:bool)
      n175 = case shown="True" w15 {
        tunnel: [w20 w30] -> w14
        tunnel: w11 -> [w20 w22]
        frame False {
        }
        frame True {
          n176 = Unbundle By Name(w22) -> ("source"=w21:string)
          n177 = Concatenate Strings("Something went wrong.  \n\nPlease try running this wizard again.  \n\nIf the problem persists please check the wizard settings or post on the LVH LINX Forums at: \n\nwww.labviewhacker.com/forums/linx \n\n", w21) -> (w23:string)
          n178 = call <vilib>:"Three Button Dialog.vi"("Allow user to close window? (TRUE)"=FALSE, "Right Button Text (\"Cancel\")"="LINX Forums" ("F button name (\"Cancel\")"), "Center Button Text (\"No\")"="Wizard Settings" ("F button name (\"Cancel\")"), "Left Button Text (\"Yes\")"="OK" ("Left Button Text (\"Yes\")"), "message"=w23) -> ("Which Button?"=w25:T13)  [unwired: 6 in]
          n179 = case shown="\"Center Button\"" w25 {
            tunnel: errorcluster {"status"=FALSE, "code"=0, "source"=""} ("error constant") -> [w32 w34 w40]
            tunnel: [w32 w33 w39] -> w30
            frame "Left Button", Default {
              # "Nothing To Do Here"
            }
            frame "Right Button" {
              w35 = "LVH-LINX"  # Campaign Source
              w36 = "In LabVIEW"  # Campaign Name
              w37 = "Firmware Wizard"  # Campaign Medium
              w38 = "www.labviewhacker.com/forums/linx"  # URL
              # "Visit Forums"
              n180 = call <vilib>:"Open Google Campaign URL.vi"("Campaign Medium"=w37, "Error In"=w34, "Campaign Source"=w35, "Campaign Name"=w36, "URL"=w38) -> ("Error Out"=w33:errorcluster)  [unwired: 5 in, 1 out]
            }
            frame "Center Button" {
              n181 = call "Firmware Wizard Config.vi"("Error In"=w40) -> ("Error Out"=w39:errorcluster)  [unwired: 10 in]
            }
          }
        }
      }
      n182 = control-ref of="This VI"() -> (w13:refnum<vi>)
      n183 = call <vilib>:"Close FP.vi"("Error In"=w14, "VI Ref"=w13) -> ("Error Out"=w12:errorcluster)  [unwired: 9 in]
      n184 = Merge Errors(w12, w11) -> (→"Error Out":errorcluster)
    }
  }
